vi "Error Cluster From Error Code.vi"(4 "is warning? (False)":bool, 5 "show call chain? (False)":bool, 6 "error in (no error)":errorcluster, 8 "error message (\"\")":string, 9 "error code (0)":i32) -> (0 "error out":errorcluster)   [LabVIEW 2014]
doc: "Converts an error or warning code to an error cluster. This VI is useful when you receive a return value from a shared library call or when you return user-defined error codes."
panel:
  in  "call chain header":string="\n<b>Complete call chain:</b>"
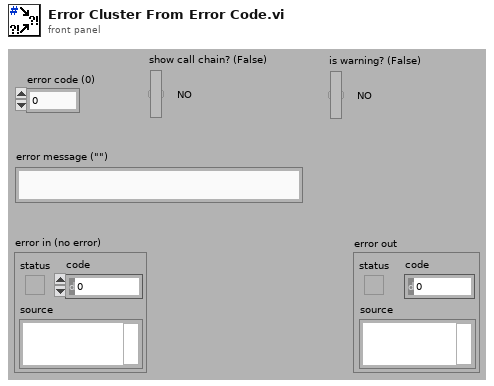
[diagram p1: front panel]
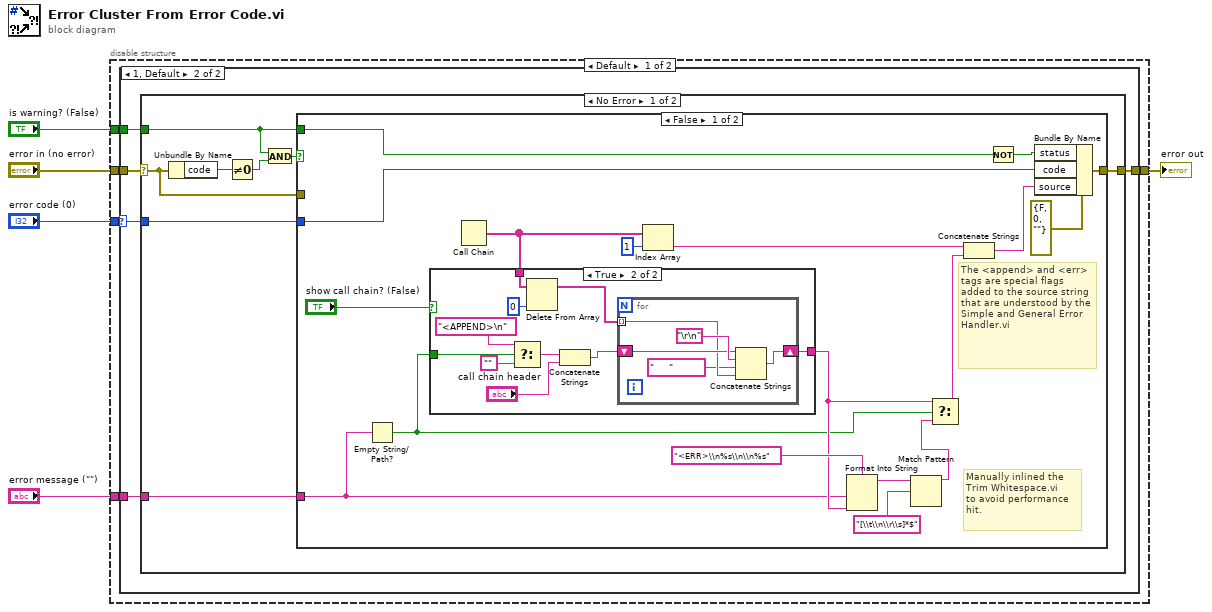
[diagram p0: block diagram]
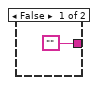
[diagram p3: hidden frame]
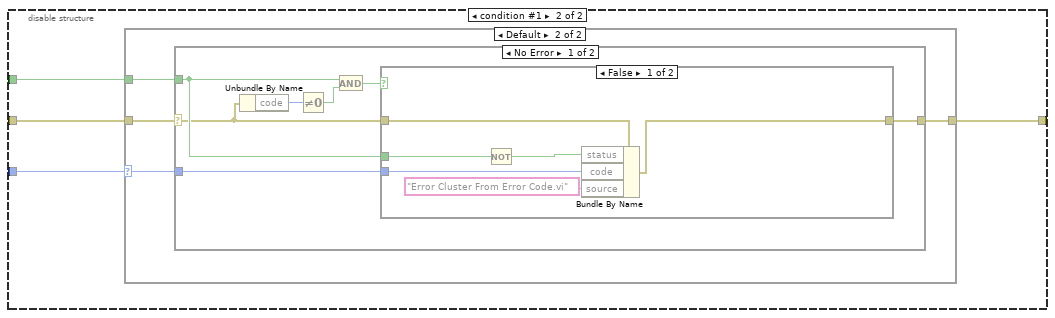
[diagram p6: hidden frame]
diagram:
  n1 = disable-structure shown="Default" {
    disable-tunnel: [w10 w63] -> w5
    disable-tunnel: "error in (no error)" -> [w9 w64]
    disable-tunnel: "error code (0)" -> [w8 w62]
    disable-tunnel: "error message (\"\")" -> [w7 _]
    disable-tunnel: "is warning? (False)" -> [w6 w61]
    frame condition #0 (active) {
      n2 = case shown="1, Default" w8 {
        selector: w8 -> [_ w14]
        tunnel: [w11 w16] -> w10
        tunnel: w9 -> [w11 w15]
        tunnel: w7 -> [_ w13]
        tunnel: w6 -> [_ w12]
        frame 0 {
          # "If the error code in equals zero, then propagate the error in cluster regardless of its value."
        }
        frame 1, Default {
          n3 = case shown="No Error" w15 {
            selector: w15 -> [w19 w60]
            tunnel: [w24 w60] -> w16
            tunnel: w14 -> [w23 _]
            tunnel: w13 -> [w18 _]
            tunnel: w12 -> [w17 _]
            frame No Error {
              n4 = Unbundle By Name(w19) -> ("code"=w22:i32)
              n5 = Not Equal To 0?(x=w22) -> (x != 0?=w20:bool)
              n6 = And(x=w17, y=w20) -> (x .and. y?=w21:bool)
              n7 = case shown="False" w21 {
                tunnel: [w42 w59] -> w24
                tunnel: w23 -> [w38 _]
                tunnel: w19 -> [_ w59]
                tunnel: w17 -> [w35 _]
                tunnel: w18 -> [w30 _]
                frame False {
                  # "Manually inlined the\nTrim Whitespace.vi\nto avoid performance\nhit."
                  # "The <append> and <err> tags are special flags added to the source string that are understood by the Simple and General Error Handler.vi"
                  n8 = Empty String/Path?(string/path=w30) -> (empty?=w29:bool)
                  n9 = Call Chain() -> (call chain=w36:string[])
                  n10 = case shown="True" "show call chain? (False)" {
                    tunnel: ["" w53] -> w32
                    tunnel: w36 -> [_ w51]
                    tunnel: w29 -> [_ w47]
                    frame False {
                    }
                    frame True {
                      n11 = Select(t="<APPEND>\n", s=w47, f="") -> (s? t:f=w44:string)
                      n12 = Delete From Array(array=w51, index=0) -> (array with subset deleted=w50:string[])  [unwired: 1 in, 1 out]
                      n13 = Concatenate Strings(w44, "call chain header") -> (w48:string)
                      n14 = for {
                        tunnel: w50 -> [w55] mode=indexing
                        shift-right: [w58] -> w53
                        shift-left: w48 -> [w56]
                        n15 = Concatenate Strings(w56, "\r\n", "     ", w55) -> (w58:string)
                      }
                    }
                  }
                  n16 = Index Array(array=w36, index=1) -> (element=w25:string)
                  n17 = Format Into String(format string="<ERR>\\n%s\\n\\n%s", w30, w32) -> (resulting string=w27:string)  [unwired: 2 in, 1 out]
                  n18 = Match Pattern(string=w27, regular expression="[\\t\\n\\r\\s]*$") -> (before substring=w26:string)  [unwired: 1 in, 3 out]
                  n19 = Select(t=w32, s=w29, f=w26) -> (s? t:f=w31:string)
                  n20 = Concatenate Strings(w25, w31) -> (w40:string)
                  n21 = Not(x=w35) -> (.not. x?=w39:bool)
                  n22 = Bundle By Name(cluster=errorcluster {"status"=FALSE, "code"=0, "source"=""} ("error out"), "status"=w39, "code"=w38, "source"=w40) -> (w42:errorcluster)
                }
                frame True {
                  # "If the error code input is setting a warning, and a warning is already set on the wire, then we\ngo with the one already on the wire."
                }
              }
            }
            frame Error {
              # "An error in trumps any error code input."
            }
          }
        }
      }
    }
    frame condition #1 {
      n23 = case shown="Default" w62 {
        selector: w62 -> [_ w67]
        tunnel: w64 -> [w65 w69]
        tunnel: [w65 w68] -> w63
        tunnel: w61 -> [_ w66]
        frame 0 {
          # "If the error code in equals zero, then propagate the error in cluster regardless of its value."
        }
        frame Default {
          n24 = case shown="No Error" w69 {
            selector: w69 -> [w71 w84]
            tunnel: [w75 w84] -> w68
            tunnel: w67 -> [w76 _]
            tunnel: w66 -> [w72 _]
            frame No Error {
              n25 = Unbundle By Name(w71) -> ("code"=w74:i32)
              n26 = Not Equal To 0?(x=w74) -> (x != 0?=w73:bool)
              n27 = And(x=w72, y=w73) -> (x .and. y?=w70:bool)
              n28 = case shown="False" w70 {
                tunnel: w76 -> [w82 _]
                tunnel: [w79 w83] -> w75
                tunnel: w72 -> [w78 _]
                tunnel: w71 -> [w77 w83]
                frame False {
                  n29 = Not(x=w78) -> (.not. x?=w81:bool)
                  n30 = Bundle By Name(cluster=w77, "status"=w81, "code"=w82, "source"="Error Cluster From Error Code.vi") -> (w79:errorcluster)
                }
                frame True {
                  # "If the error code input is setting a warning, and a warning is already set on the wire, then we\ngo with the one already on the wire."
                }
              }
            }
            frame Error {
              # "An error in trumps any error code input."
            }
          }
        }
      }
    }
  }
  "error out" <- w5
